vi "CenterPoint.vi"(8 "error in (no error)":errorcluster, 11 "PointSpecialized in":refnum<class "PointSpecialized.lvclass">) -> (0 "error out":errorcluster, 2 "CenterPoint":refnum<class "Point.lvclass">, 3 "PointSpecialized out":refnum<class "PointSpecialized.lvclass">)   [LabVIEW 2021, in "Picture2D.lvlib" / "PointSpecialized.lvclass"]
uses:
  PointSpecialized.lvclass
  C:/Users/Dany/OneDrive/LabVIEW/Class/Picture2D/Point/Point.lvclass
  Point/Point.lvclass
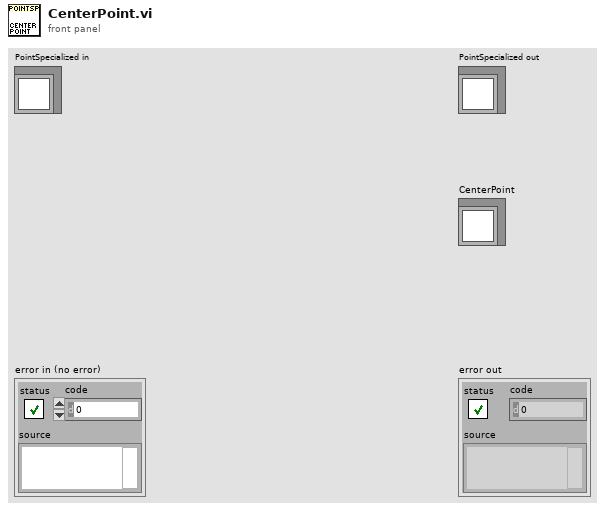
[diagram p1: front panel]
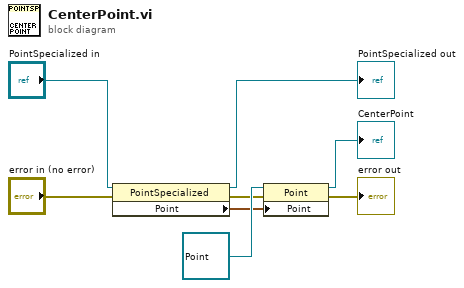
[diagram p0: block diagram]
diagram:
  n1 = property class="PointSpecialized"(reference="PointSpecialized in", error in="error in (no error)") -> (reference out=→"PointSpecialized out":refnum<class "PointSpecialized.lvclass">, error out=w2:errorcluster, "Point"=w4:cluster{"x":i16, "y":i16})
  n2 = property class="Point"(reference=refnum<class "Point.lvclass"> refnum ("CenterPoint"), error in=w2, "Point"=w4) -> (reference out=→"CenterPoint":refnum<class "Point.lvclass">, error out=→"error out":errorcluster)
